vi "Update_Booking_MCODE.vi"(8 "error in (no error)":errorcluster, 10 "Bootout":T2 {"End Time" format="%<%d/%m/%Y\n%I:%M:%S %p>T"; "Start Time" format="%<%d/%m/%Y\n%I:%M:%S %p>T"}, 11 "Ref in":T4={"MS SQL Connection"=refnum, "UDL File"=path "", "Time"="", "DCODE"="", "WIP+1"=0, "MC No?"=0, "POKAYOKE?"=FALSE, "Expected Result"="", "Result [Status]"="", "Clock"=0.0, "RFID"="", "WIP Queue"=refnum, "TS Parameter"={"ProfitCenterCode"="", "LineCode"="", "WorkOrderNumber"="", "Model"="", "Model_with_Prefix"="", "VendorCode"="", "SetParameterDateCode"="", "PokaYoke"=0, "Target"=1, "Live_DateCode"="", "CustomerPartNumber"="", "Hand"="", "sBarcode"=FALSE, "FCA"=0, "Ent_Stamp"=timestamp(0 s since 1904-01-01), "STS_CD"=0.0}, "Data_Queue"=[], "RFID Serial No."=""} {"TS Parameter"."FCA" format="%01d"; "TS Parameter"."Target" min=1 max=100000; "TS Parameter"."PokaYoke" min=0 max=1}) -> (0 "error out":errorcluster, 3 "Ref out":T4={"MS SQL Connection"=refnum, "UDL File"=path "", "Time"="", "DCODE"="", "WIP+1"=0, "MC No?"=0, "POKAYOKE?"=FALSE, "Expected Result"="", "Result [Status]"="", "Clock"=0.0, "RFID"="", "WIP Queue"=refnum, "TS Parameter"={"ProfitCenterCode"="", "LineCode"="", "WorkOrderNumber"="", "Model"="", "Model_with_Prefix"="", "VendorCode"="", "SetParameterDateCode"="", "PokaYoke"=0, "Target"=1, "Live_DateCode"="", "CustomerPartNumber"="", "Hand"="", "sBarcode"=FALSE, "FCA"=0, "Ent_Stamp"=timestamp(0 s since 1904-01-01), "STS_CD"=0.0}, "Data_Queue"=[], "RFID Serial No."=""} {"TS Parameter"."FCA" format="%01d"; "TS Parameter"."Target" min=1 max=100000; "TS Parameter"."PokaYoke" min=0 max=1})   [LabVIEW 2020]
uses:
  Controls/TD SQL.ctl
  <vilib>/addons/database/Connection.llb/Conn ObjectReference.ctl
  Controls/WIP_State.ctl
  Controls/TS_Parameter.ctl
  Controls/Breakdown_List.ctl
  Controls/Loss_type.ctl
  MS SQL/MS_Global.vi
  <vilib>/addons/database/NI_Database_API.lvlib
panel:
  out "resulting string":string
  out "Machine":T1(ring)
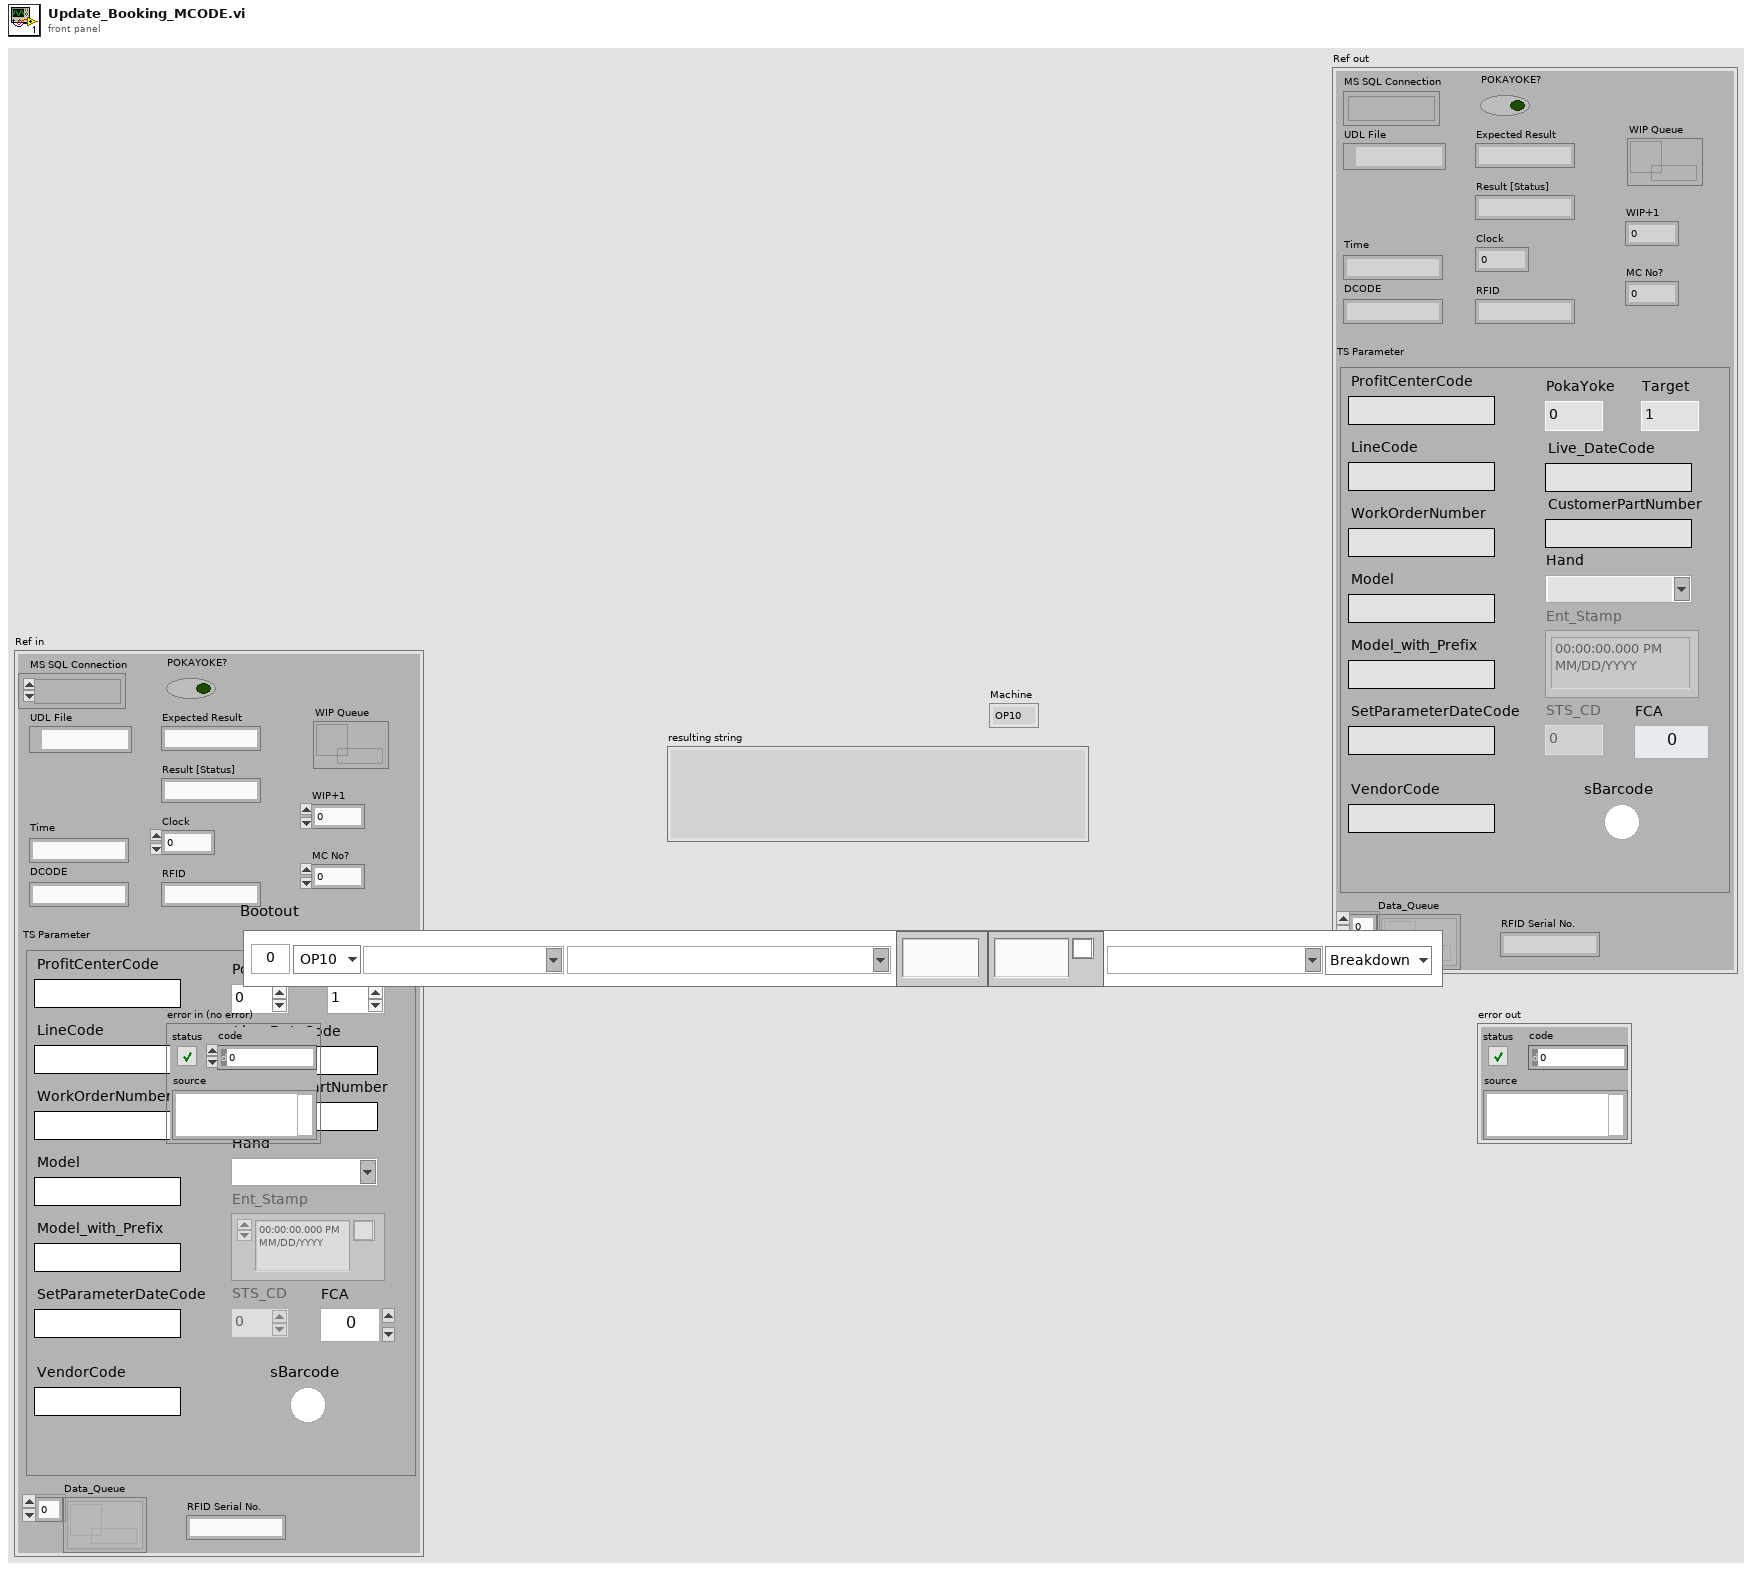
[diagram p1: front panel]
types:
  T1 = enum16{"OP10", "OP20", "OP30", "OP40", "OP50", "OP60", "OP70", "OP80", "LINE"}
  T2 = typedef "Breakdown_List.ctl" = cluster{"S.No":i32, "Reason Code":string, "Start Time":timestamp, "End Time":timestamp, "Operator":string, "Type":T3, "Machine":enum16{"OP10", "OP20", "OP30", "OP40", "OP50", "OP60", "OP70", "OP80", "LINE"}, "Reason":string}
  T3 = typedef "Loss_type.ctl" = enum16{"Breakdown", "Bookout"}
  T4 = typedef "TD SQL.ctl" = cluster{"MS SQL Connection":T5, "UDL File":path, "Time":string, "DCODE":string, "WIP+1":i64, "MC No?":i32, "POKAYOKE?":bool, "Expected Result":string, "Result [Status]":string, "Clock":dbl, "RFID":string, "WIP Queue":refnum<queue>, "TS Parameter":T6, "Data_Queue":refnum<queue>[], "RFID Serial No.":string}
  T5 = typedef "NI_Database_API.lvlib/Conn ObjectReference.ctl" = refnum<k1>
  T6 = typedef "TS_Parameter.ctl" = cluster{"ProfitCenterCode":string, "LineCode":string, "WorkOrderNumber":string, "Model":string, "Model_with_Prefix":string, "VendorCode":string, "SetParameterDateCode":string, "PokaYoke":i32, "Target":i32, "Live_DateCode":string, "CustomerPartNumber":string, "Hand":string, "sBarcode":bool, "FCA":i32, "Ent_Stamp":timestamp, "STS_CD":dbl}
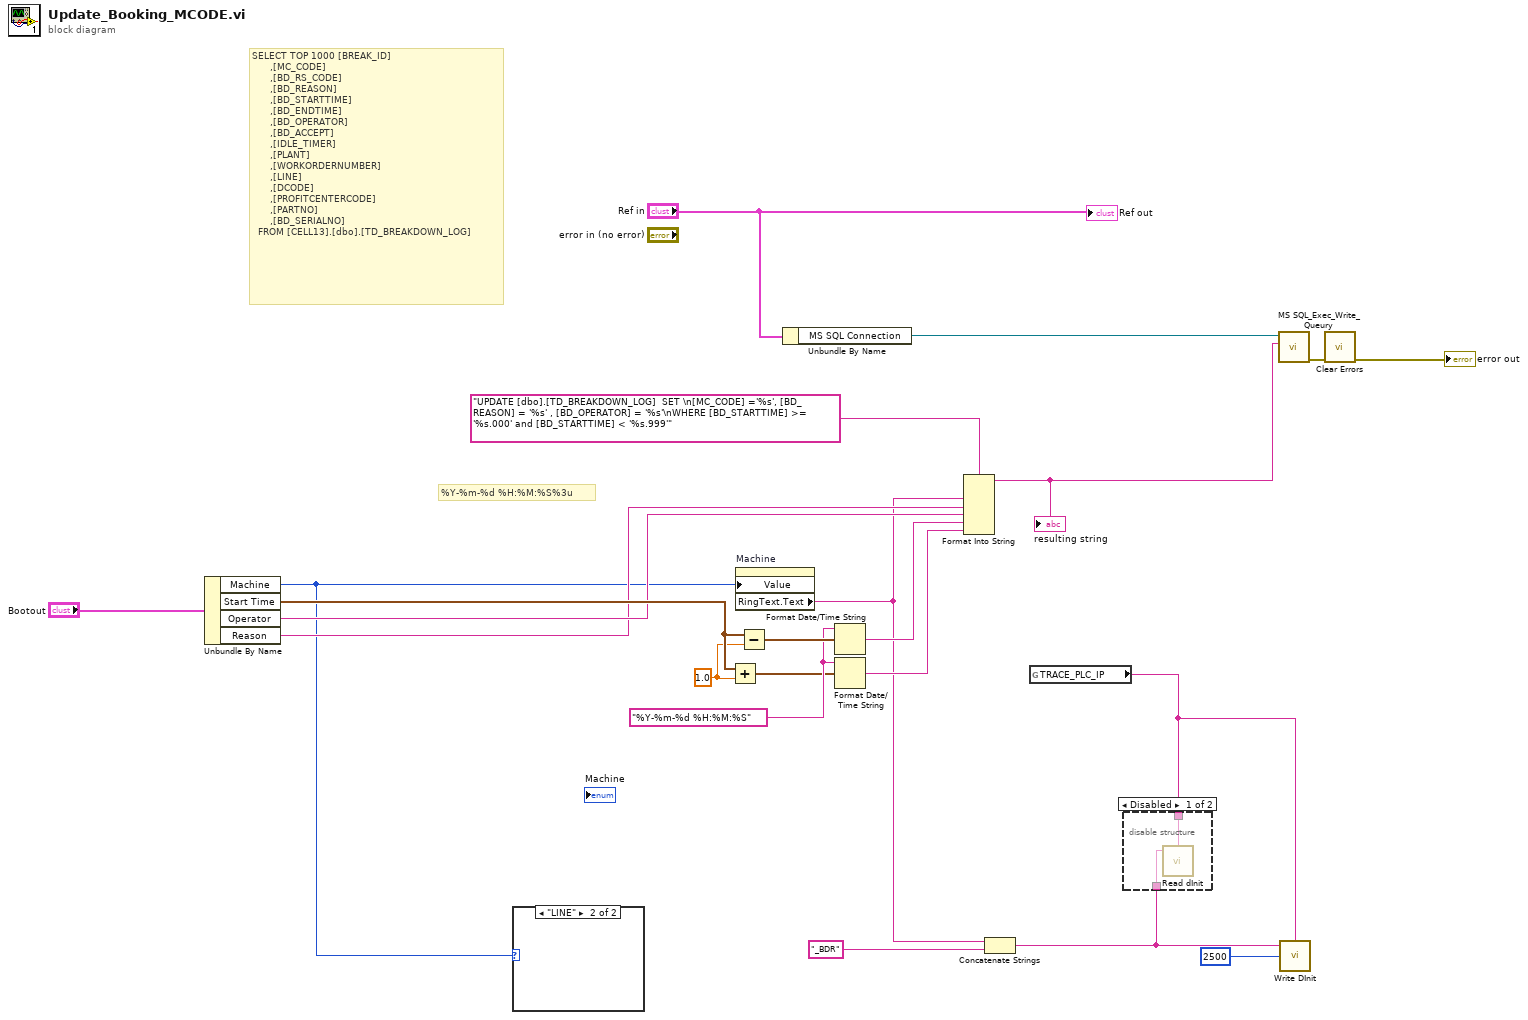
[diagram p0: block diagram]
diagram:
  w13 = 1.0 ("y")
  w12 = "%Y-%m-%d %H:%M:%S" ("time format string (%c)")
  # "%Y-%m-%d %H:%M:%S%3u"
  # "SELECT TOP 1000 [BREAK_ID]\n      ,[MC_CODE]\n      ,[BD_RS_CODE]\n      ,[BD_REASON]\n      ,[BD_STARTTIME]\n      ,[BD_ENDTIME]\n      ,[BD_OPERATOR]\n      ,[BD_ACCEPT]\n      ,[IDLE_TIMER]\n      ,[PLANT]\n      ,[WORKORDERNUMBER]\n      ,[LINE]\n      ,[DCODE]\n      ,[PROFITCENTERCODE]\n      ,[PARTNO]\n      ,[BD_SERIALNO]\n  FROM [CELL13].[dbo].[TD_BREAKDOWN_LOG]"
  n1 = Unbundle By Name("Bootout") -> ("Machine"=w5:T1, "Start Time"=w14:timestamp, "Operator"=w8:string, "Reason"=w7:string)
  n2 = case shown="\"LINE\"" w5 {
    frame "OP10", Default {
    }
    frame "LINE" {
    }
  }
  n3 = Add(x=w14, y=w13) -> (x+y=w11:timestamp)
  n4 = property on="Machine" class="Enum (strict)"("Value"=w5) -> ("RingText.Text"=w4:string)  [unwired: 2 in, 2 out]
  n5 = Subtract(x=w14, y=w13) -> (x-y=w15:timestamp)
  n6 = Unbundle By Name("Ref in") -> ("MS SQL Connection"=w21:T5)
  n7 = Format Date/Time String(time format string (%c)=w12, seconds (now)=w15) -> (date/time string=w10:string)  [unwired: 1 in]
  n8 = Format Date/Time String(time format string (%c)=w12, seconds (now)=w11) -> (date/time string=w9:string)  [unwired: 1 in]
  n9 = Format Into String(format string="UPDATE [dbo].[TD_BREAKDOWN_LOG]  SET \n[MC_CODE] ='%s', [BD_REASON] = '%s' , [BD_OPERATOR] = '%s'\nWHERE [BD_STARTTIME] >= '%s.000' and [BD_STARTTIME] < '%s.999'" ("Operator"), w4, w7, w8, w10, w9) -> (resulting string=w18:string)  [unwired: 2 in, 1 out]
  "resulting string" <- w18
  n10 = Concatenate Strings(w4, "_BDR" ("String")) -> (w2:string)
  n11 = global read "MS_Global.vi" "TRACE_PLC_IP"() -> (w1:string)
  n12 = disable-structure shown="Disabled" {
    disable-tunnel: w2 -> [w24 _]
    disable-tunnel: w1 -> [w23 _]
    frame Disabled {
      n13 = call "Read dInit.vi"("Network Path"=w23, "Tag Name"=w24) -> ()  [unwired: 3 in, 1 out]
    }
    frame Enabled {
    }
  }
  n14 = call "MS SQL_Exec_Write_Queury.vi"("Query"=w18, "Refnum in"=w21) -> ("error out"=w17:errorcluster)  [unwired: 8 in, 1 out]
  n15 = call "Write DInit.vi"("Network Path"=w1, "Int"=2500, "Tag Name"=w2) -> ()  [unwired: 2 in]
  n16 = call <vilib>:"Clear Errors.vi"("error in (no error)"=w17) -> ("error out"=→"error out":errorcluster)  [unwired: 5 in, 1 out]
  "Ref out" <- "Ref in"
